vi "WriteSingleCoil.vi"(0 "VISA Refnum in":refnum<visa-resource-name>, 5 "Cluster":T1, 7 "Coil":u16, 9 "Coil Value":bool, 11 "error in":errorcluster, 12 "Enable":bool) -> (4 "VISA out":refnum<visa-resource-name>, 6 "Cluster Out":T1, 15 "error out":errorcluster)   [LabVIEW 2020]
uses:
  <vilib>/NI Modbus.llb/MB Serial Master Query Write Single Coil (poly).vi
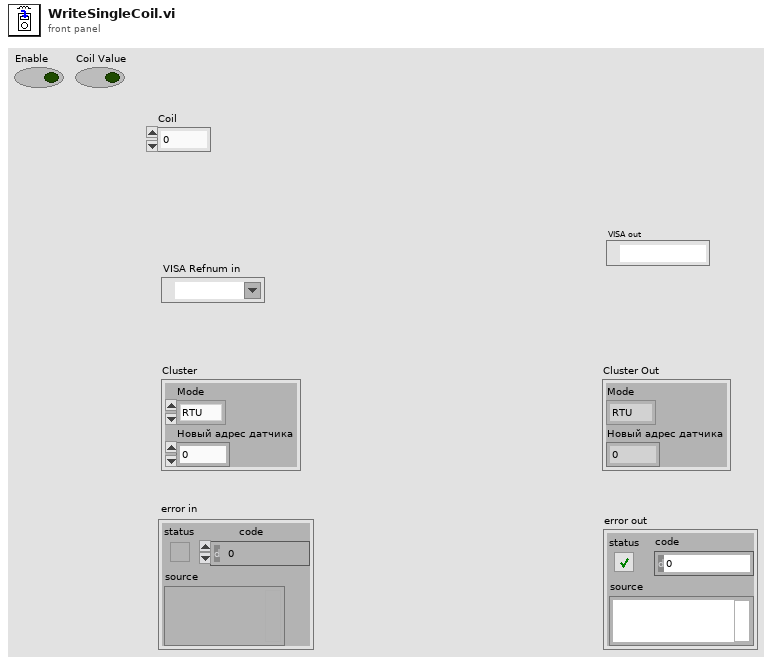
[diagram p1: front panel]
types:
  T1 = cluster{"Mode":enum16{"RTU", "ASCII"}, "Новый адрес датчика":u16}
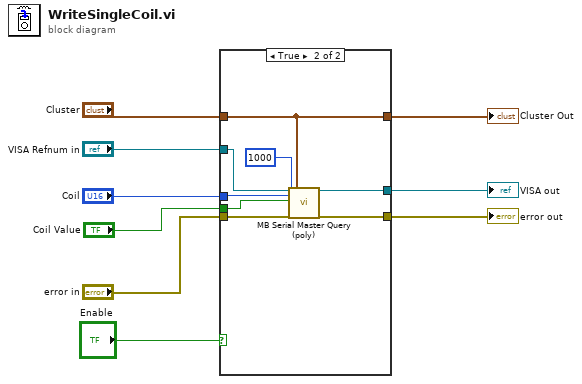
[diagram p0: block diagram]
diagram:
  n1 = case shown="True" "Enable" {
    tunnel: "VISA Refnum in" -> [w10 w20]
    tunnel: "error in" -> [w12 w19]
    tunnel: "Coil" -> [_ w14]
    tunnel: [w10 w18] -> w7
    tunnel: [w12 w17] -> w6
    tunnel: "Cluster" -> [w11 w16]
    tunnel: [w11 w16] -> w3
    tunnel: "Coil Value" -> [_ w13]
    frame False {
    }
    frame True {
      n2 = call-poly <vilib>:"MB Serial Master Query (poly).vi"("VISA resource name"=w20, "Address"=w14, "Coil"=w13, "Timeout"=u32 1000, "error in"=w19, "Serial Parameters"=w16) -> ("VISA resource name out"=w18:refnum<visa-resource-name>, "error out"=w17:errorcluster)  [unwired: 11 in, 1 out]
    }
  }
  "error out" <- w6
  "VISA out" <- w7
  "Cluster Out" <- w3
